vi "Get Year Month Day and Seconds UUID-value lists.vi"() -> (0 "values":dbl[](array[numeric]), 1 "UUIDs":string[](array[string]))   [LabVIEW 2020]
doc: "Returns the UUID-values lists for the year, month, day, and time in seconds from midnight."
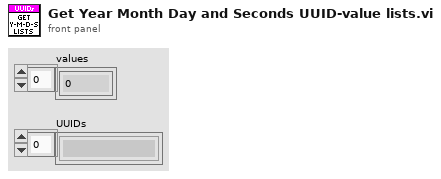
[diagram p1: front panel]
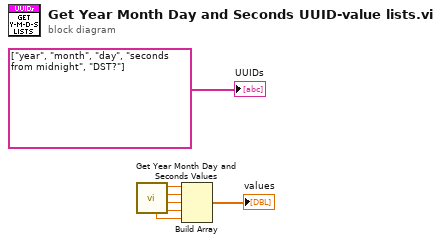
[diagram p0: block diagram]
diagram:
  n1 = call "Get Year Month Day and Seconds Values.vi"() -> ("seconds from 00:00"=w5:dbl, "day"=w4:dbl, "month"=w3:dbl, "year"=w2:dbl, "DST?"=w1:dbl)  [unwired: 5 in, 2 out]
  n2 = Build Array(w2, w3, w4, w5, w1) -> (→"values":dbl[])
  "UUIDs" <- string[] ["year", "month", "day", "seconds from midnight", "DST?"]
